vi "Clear.vi"(8 "error in (no error)":errorcluster, 11 "Mixer in":refnum<class "Mixer.lvclass">) -> (0 "error out":errorcluster, 2 "Audio Device":T1, 3 "Mixer out":refnum<class "Mixer.lvclass">)   [LabVIEW 2020, in "G-Audio.lvlib" / "Mixer.lvclass"]
uses:
  Mixer.lvclass
  Controls/Audio Device Refnum.ctl
  Mixer.lvclass/Mixer.ctl
  Channel/Channel.lvclass
  G-Audio.lvlib
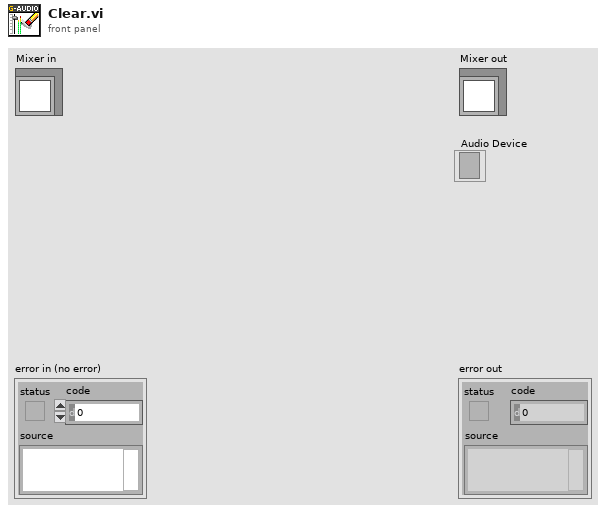
[diagram p1: front panel]
types:
  T1 = typedef "G-Audio.lvlib/Audio Device Refnum.ctl" = refnum<file>
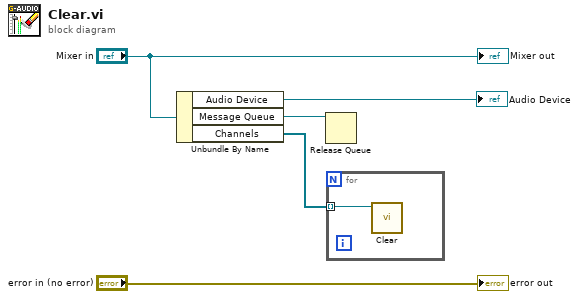
[diagram p0: block diagram]
diagram:
  n1 = Unbundle By Name("Mixer in") -> ("Audio Device"=→"Audio Device":T1, "Message Queue"=w3:refnum<queue>, "Channels"=w2:refnum<data-value>[])
  n2 = Release Queue(queue=w3) -> ()  [unwired: 2 in, 3 out]
  n3 = for {
    tunnel: w2 -> [w6] mode=indexing
    n4 = call "Clear.vi"("Channel in"=w6) -> ()  [unwired: 10 in, 1 out]
  }
  "error out" <- "error in (no error)"
  "Mixer out" <- "Mixer in"
